vi "Function.vi"(8 "error in (no error)":errorcluster, 10 "Value":dbl, 11 "Two Terminal in":refnum<class "Reciprocal_CPLX_EXT.lvclass">) -> (0 "error out":errorcluster, 2 "Result":dbl, 3 "Two Terminal out":refnum<class "Reciprocal_CPLX_EXT.lvclass">)   [LabVIEW 2021, in "Reciprocal_CPLX_EXT.lvclass"]
uses:
  Reciprocal_CPLX_EXT.lvclass
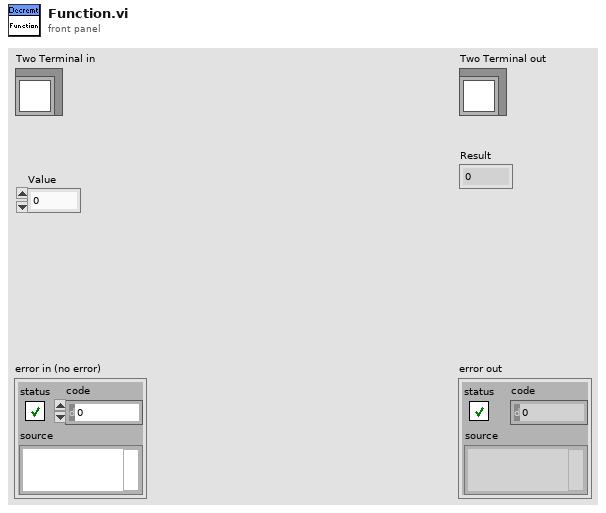
[diagram p1: front panel]
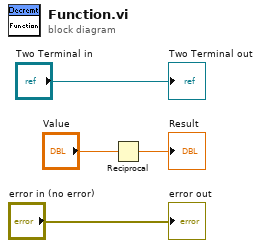
[diagram p0: block diagram]
diagram:
  n1 = Reciprocal(x="Value") -> (1/x=→"Result":dbl)
  "error out" <- "error in (no error)"
  "Two Terminal out" <- "Two Terminal in"
